vi "FGV FT-IR Kuehler.vi"(6 "Aktionen":T1, 7 "N2 zu PNS":u16, 8 "FT-IR Kühler":u16, 9 "Durchflusssensor 0-5V":u16, 10 "LN2 Spülen":u16, 11 "mit GN2 spülen":u16) -> (0 "FT-IR Kühler":u16, 1 "Durchflusssensor 0-5V":bool, 2 "LN2 Spülen":bool, 3 "mit GN2 spülen":bool, 5 "N2 zu PNS":bool)   [LabVIEW 2020, in "Allgemein.lvlib"]
uses:
  Allgemein.lvlib
  FGV FT-IR Kuehlung Aktionen.ctl
panel:
  # "0 = aktiv\n1 = inaktiv"
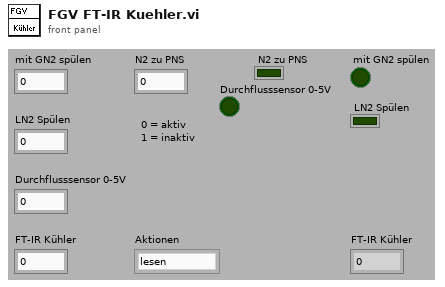
[diagram p1: front panel]
types:
  T1 = typedef "Allgemein.lvlib/FGV FT-IR Kuehlung Aktionen.ctl" = enum16{"lesen", "Kühlung?"}
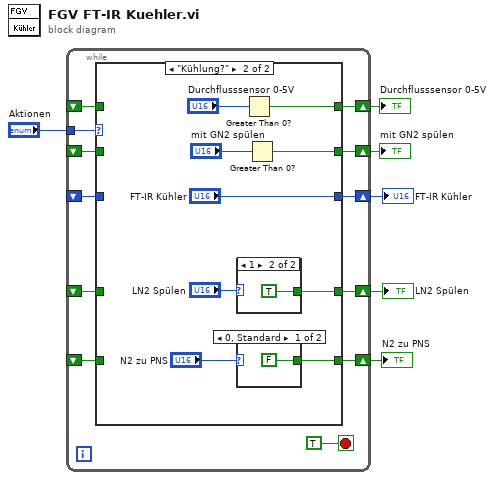
[diagram p0: block diagram]
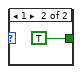
[diagram p3: hidden frame]
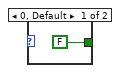
[diagram p4: hidden frame]
diagram:
  n1 = while {
    tunnel: "Aktionen" -> [w17]
    shift-right: [w15] -> w5
    shift-left: _ -> [w16]
    shift-right: [w14] -> w4
    shift-left: _ -> [w13]
    shift-right: [w12] -> w2
    shift-left: _ -> [w11]
    shift-right: [w10] -> w1
    shift-left: _ -> [w9]
    shift-right: [w8] -> w3
    shift-left: _ -> [w7]
    stop <- TRUE stop-if-true
    n2 = case shown="\"Kühlung?\"" w17 {
      tunnel: w16 -> [w23 _]
      tunnel: [w23 "FT-IR Kühler"] -> w15
      tunnel: [w22 w30] -> w14
      tunnel: w13 -> [w22 _]
      tunnel: [w21 w26] -> w12
      tunnel: w11 -> [w21 _]
      tunnel: [w20 w24] -> w10
      tunnel: w9 -> [w20 _]
      tunnel: [w19 w28] -> w8
      tunnel: w7 -> [w19 _]
      frame "lesen", Default {
      }
      frame "Kühlung?" {
        n3 = case shown="1" "LN2 Spülen" {
          tunnel: [FALSE TRUE] -> w30
          frame 0, Default {
          }
          frame 1 {
          }
        }
        n4 = case shown="0, Standard" "N2 zu PNS" {
          tunnel: [FALSE TRUE] -> w28
          frame 0, Default {
          }
          frame 1 {
          }
        }
        n5 = Greater Than 0?(x="Durchflusssensor 0-5V") -> (x > 0?=w24:bool)
        n6 = Greater Than 0?(x="mit GN2 spülen") -> (x > 0?=w26:bool)
      }
    }
  }
  "FT-IR Kühler" <- w5
  "LN2 Spülen" <- w4
  "N2 zu PNS" <- w3
  "mit GN2 spülen" <- w2
  "Durchflusssensor 0-5V" <- w1
